vi "Detector.vi"() -> ()   [LabVIEW 2018]
panel:
  out "XZ Graph":cluster{dbl[], dbl[]}(graph)
  in  "velocity":dbl
  out "vZinitial":dbl
  out "vXinitial":dbl
  out "timeOfFlight":dbl format="%#_5g"
  in  "bField":dbl
  in  "height":dbl
  out "vYinitial":dbl
  in  "eField":dbl
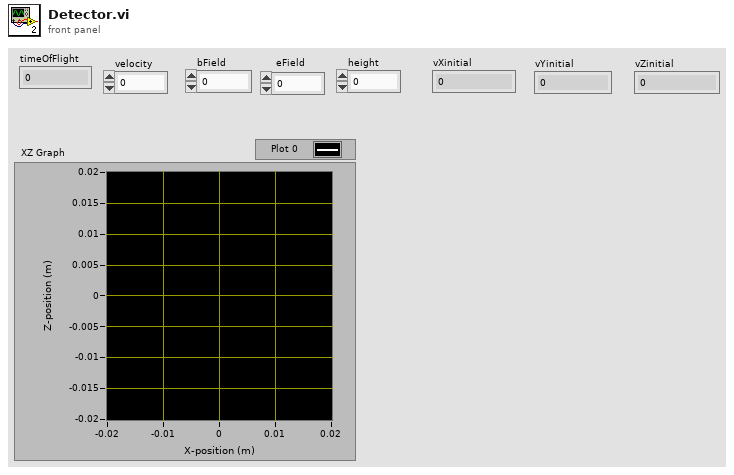
[diagram p1: front panel]
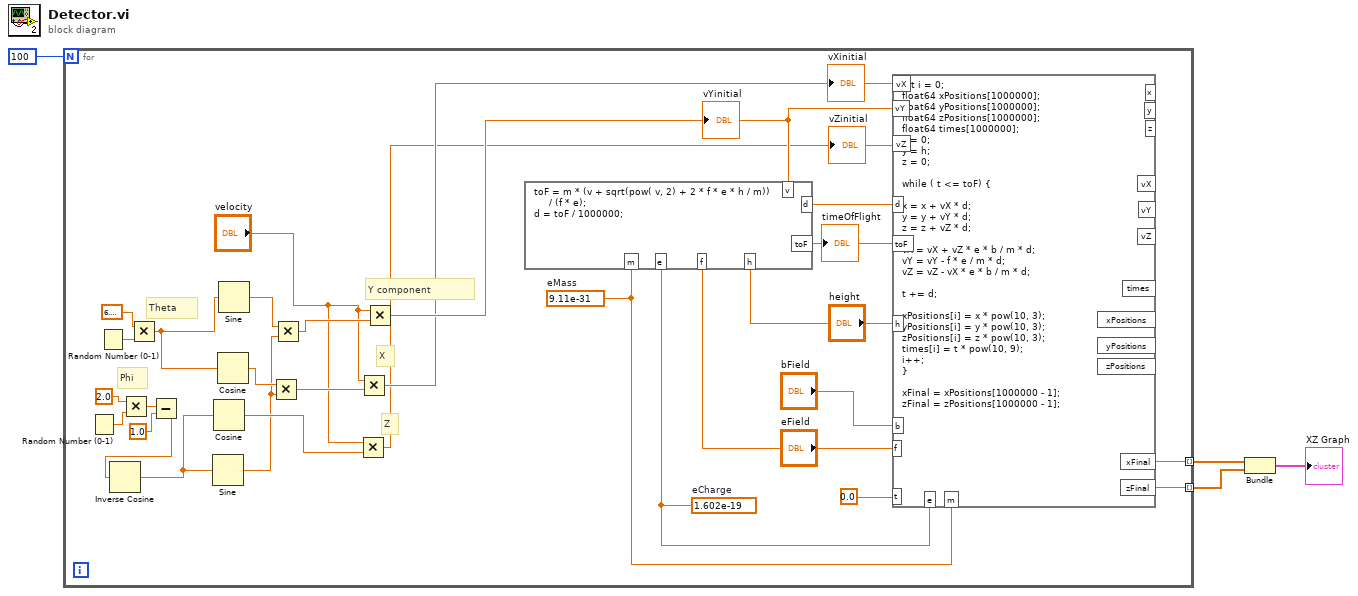
[diagram p0: block diagram]
diagram:
  n1 = for {
    N: 100 -> [_]
    tunnel: [w6] -> w4 mode=indexing
    tunnel: [w5] -> w3 mode=indexing
    w31 = 1.602e-19  # eCharge
    w30 = 9.11e-31  # eMass
    # "Phi"
    # "Theta"
    # "Z"
    # "X"
    # "Y component"
    n2 = Random Number (0-1)() -> (number: 0 to 1=w22:dbl)
    n3 = Random Number (0-1)() -> (number: 0 to 1=w25:dbl)
    n4 = Multiply(x=2.0, y=w22) -> (x*y=w21:dbl)
    n5 = Multiply(x=6.283185307179586, y=w25) -> (x*y=w19:dbl)
    n6 = Subtract(x=w21, y=1.0) -> (x-y=w18:dbl)
    n7 = Inverse Cosine(1:w18) -> (0:w17:dbl)
    n8 = Sine(x=w17) -> (sin(x)=w12:dbl)
    n9 = Cosine(x=w17) -> (cos(x)=w16:dbl)
    n10 = Cosine(x=w19) -> (cos(x)=w13:dbl)
    n11 = Sine(x=w19) -> (sin(x)=w15:dbl)
    n12 = Multiply(x=w13, y=w12) -> (x*y=w11:dbl)
    n13 = Multiply(x=w15, y=w12) -> (x*y=w14:dbl)
    n14 = Multiply(x="velocity", y=w16) -> (x*y=w8:dbl)
    "vZinitial" <- w8
    n15 = Multiply(x="velocity", y=w11) -> (x*y=w9:dbl)
    "vXinitial" <- w9
    n16 = Multiply(x="velocity", y=w14) -> (x*y=w10:dbl)
    "vYinitial" <- w10
    n17 = formula code="toF = m * (v + sqrt(pow( v, 2) + 2 * f * e * h / m))\n     / (f * e);\nd = toF / 1000000;"("f"="eField", "h"="height", "v"=w10, "m"=w30, "e"=w31) -> ("toF"=w28:dbl, "d"=w29:dbl)
    "timeOfFlight" <- w28
    n18 = formula code="int i = 0;\nfloat64 xPositions[1000000];\nfloat64 yPositions[1000000];\nfloat64 zPositions[1000000];\nfloat64 times[1000000];\nx = 0;\ny = h;\nz = 0;\n\nwhile ( t <= toF) {\n\nx = x + vX * d;\ny = y + vY * d;\nz = z + vZ * d;\n\nvX = vX + vZ * e * b / m * d;\nvY = vY - f * e / m * d;\nvZ = vZ - vX * e * b / m * d;\n\nt += d;\n\nxPositions[i] = x * pow(10, 3);\nyPositions[i] = y * pow(10, 3);\nzPositions[i] = z * pow(10, 3);\ntimes[i] = t * pow(10, 9);\ni++;\n}\n\nxFinal = xPositions[1000000 - 1];\nzFinal = zPositions[1000000 - 1];"("vY"=w10, "e"=w31, "m"=w30, "f"="eField", "d"=w29, "h"="height", "toF"=w28, "t"=0.0, "b"="bField", "vX"=w9, "vZ"=w8) -> ("xFinal"=w6:dbl, "zFinal"=w5:dbl)  [unwired: 10 out]
  }
  n19 = Bundle(w4, w3) -> (→"XZ Graph":cluster{dbl[], dbl[]})  [unwired: 1 in]
